vi "APC_HRLtest.vi"() -> (3 "IMEPg [bar]":dbl[](array[numeric]), 5 "IMEPn [bar]":dbl[](array[numeric]))   [LabVIEW 2020]
doc: "This example demonstrates the procedure required to apply different NI-DAQmx Custom Scales to each virtual channel in a task. A DAQmx Task Property Node (Functions >> NI Measurements >> DAQmx - Data Acquisition >> DAQmx Advanced Task Options) is used to obtain the task's virtual channels. A DAQmx Channel Property Node (Functions >> NI Measurements >> DAQmx - Data Acquisition) is then used to set the custom scale for each virtual channel in the task.\n\nThe \"DAQmx Create Scale\" VI creates a custom scale for each channel in the channel list. *Note, make sure your Minimum and Maximum channel parameters are consistent with the range the scale will create."
uses:
  <vilib>/Utility/file.llb/Write Delimited Spreadsheet (DBL).vi
panel:
  out "V [m^3]":dbl[](array[numeric])
  out "output array":dbl[](array[numeric])
  out "appended array":dbl[][](array[numeric])
  out "Waveform Graph":dbl[][](graph)
  out "HRL":dbl[][](array[numeric])
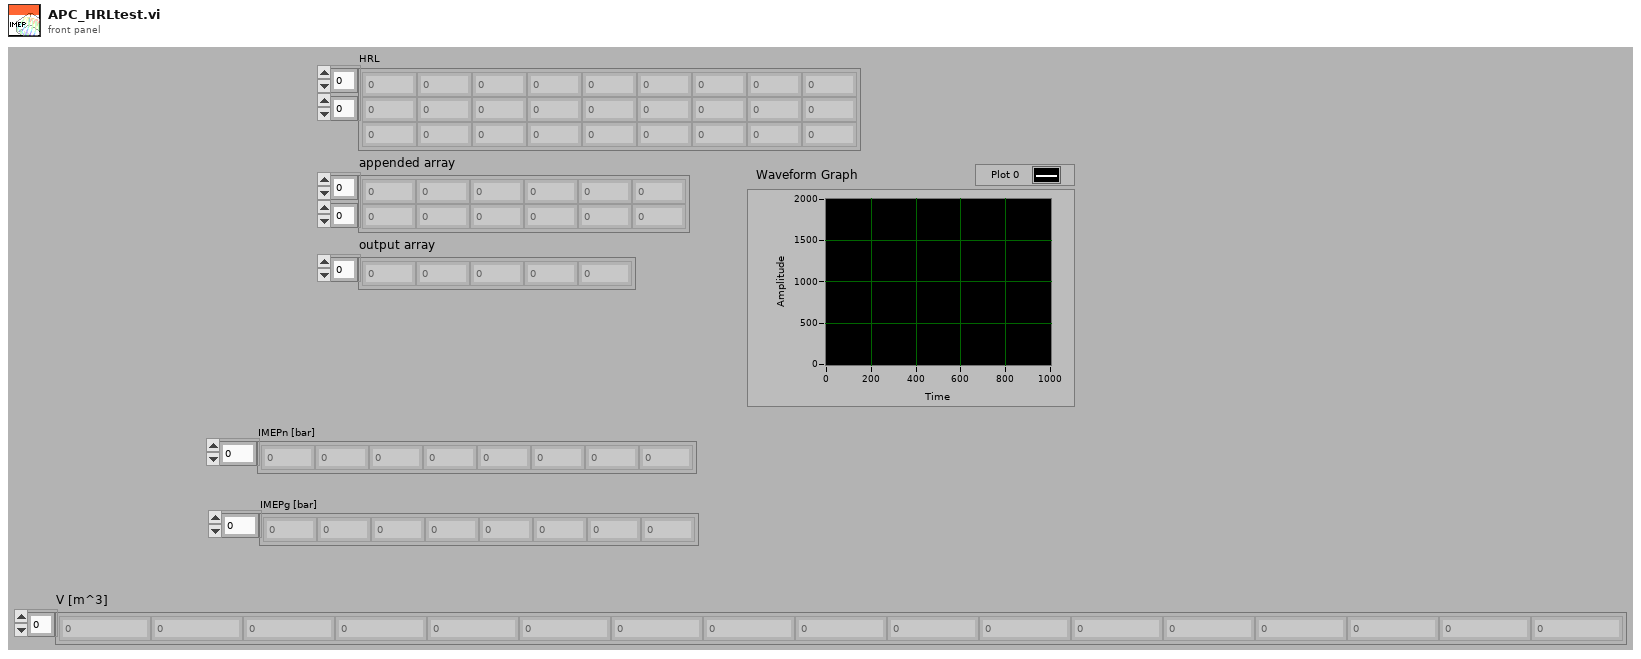
[diagram p1: front panel]
types:
  T1 = typedef "APC_volume.ctl" = cluster{"V [m^3]":dbl[], "dV [m^3/CAD]":dbl[], "Vdis [m^3]":dbl, "Surface [m^2]":dbl[], "CAD/sample":dbl}
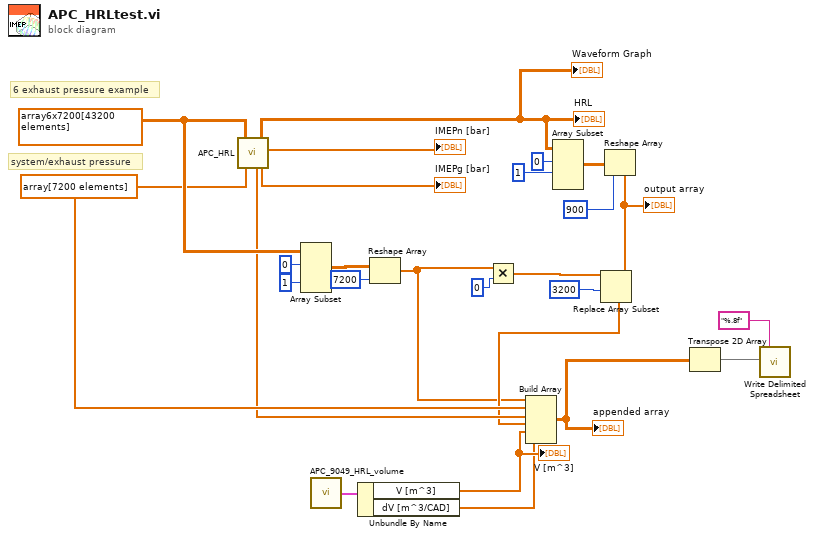
[diagram p0: block diagram]
diagram:
  w21 = dbl[] array[7200 elements] ("exhaust pressure")
  w24 = dbl[][] array6x7200[43200 elements] ("6 P cyl exmple")
  # "system/exhaust pressure"
  # "6 exhaust pressure example"
  n1 = call "APC_HRL.vi"("Pcyl"=w24, "exhaust pressure"=w21) -> ("HRL"=w15:dbl[][], "IMEPn [bar]"=→"IMEPn [bar]":dbl[], "IMEPg [bar]"=→"IMEPg [bar]":dbl[], "pegged"=w18:dbl[])
  "HRL" <- w15
  "Waveform Graph" <- w15
  n2 = Array Subset(array=w24, index (row)=0 ("index"), length (row)=1 ("length")) -> (w8:dbl[][])  [unwired: 2 in]
  n3 = call "APC_9049_HRL_volume.vi"() -> ("Volume cluster"=w4:T1)  [unwired: 2 in]
  n4 = Unbundle By Name(w4) -> ("V [m^3]"=w3:dbl[], "dV [m^3/CAD]"=w2:dbl[])
  "V [m^3]" <- w3
  n5 = Reshape Array(w8, 7200 ("dimension size")) -> (w7:dbl[])
  n6 = Multiply(x=w7, y=0 ("index")) -> (x*y=w13:dbl[])
  n7 = Array Subset(array=w15, index (row)=0 ("index"), length (row)=1 ("length")) -> (w12:dbl[][])  [unwired: 2 in]
  n8 = Reshape Array(w12, 900 ("dimension size")) -> (w10:dbl[])
  "output array" <- w10
  n9 = Replace Array Subset(array=w13, new element=w10, index=3200 ("index (row)")) -> (w9:dbl[])
  n10 = Build Array(w7, w21, w18, w9, w3, w2) -> (w20:dbl[][])
  "appended array" <- w20
  n11 = Transpose 2D Array(2D array=w20) -> (transposed array=w19:dbl[][])
  n12 = call-poly <vilib>:"Write Delimited Spreadsheet.vi"("format (%.3f)"="%.8f", "2D data"=w19) -> ()  [unwired: 12 in, 2 out]
